vi "DeleteObstacle.vi"(6 "OldVal":bool, 7 "ID# To Delete (miss)":u16, 8 "error in (no error)":errorcluster, 10 "Obstacle Arrays Cluster IN":T1 {"Readable Obstacles"."Obstacle Array"."North" format="%#_10f"; "Readable Obstacles"."Obstacle Array"."East" format="%#_8f"}, 11 "NetworkStreamWriter in":refnum<class "NetworkStreamWriter.lvclass">) -> (0 "error out":errorcluster, 2 "Obstacle Arrays Cluster OUT":T1 {"Readable Obstacles"."Obstacle Array"."North" format="%#_10f"; "Readable Obstacles"."Obstacle Array"."East" format="%#_8f"}, 3 "NetworkStreamWriter out":refnum<class "NetworkStreamWriter.lvclass">)   [LabVIEW 2013]
doc: "This VI takes the \"ID to Delete\" value and\n1) Sends that ID down to the forebrain\n2) Deletes the objects with that ID from the OCU mission arrays\n\nEric Schneider, August 2014"
uses:
  RIO-OCU_Comm/NetworkStreams/Writer/NetworkStreamWriter.lvclass
  TypeDef/obstacle_arrays.ctl
  cRIO_Code/Logic/Classes/Obstacle/Obstacle.lvclass
  cRIO_Code/Data/TypeDefs/ObstacleDescription.ctl
  cRIO_Code/Data/TypeDefs/UTM Location.ctl
  CommandMessages.ctl
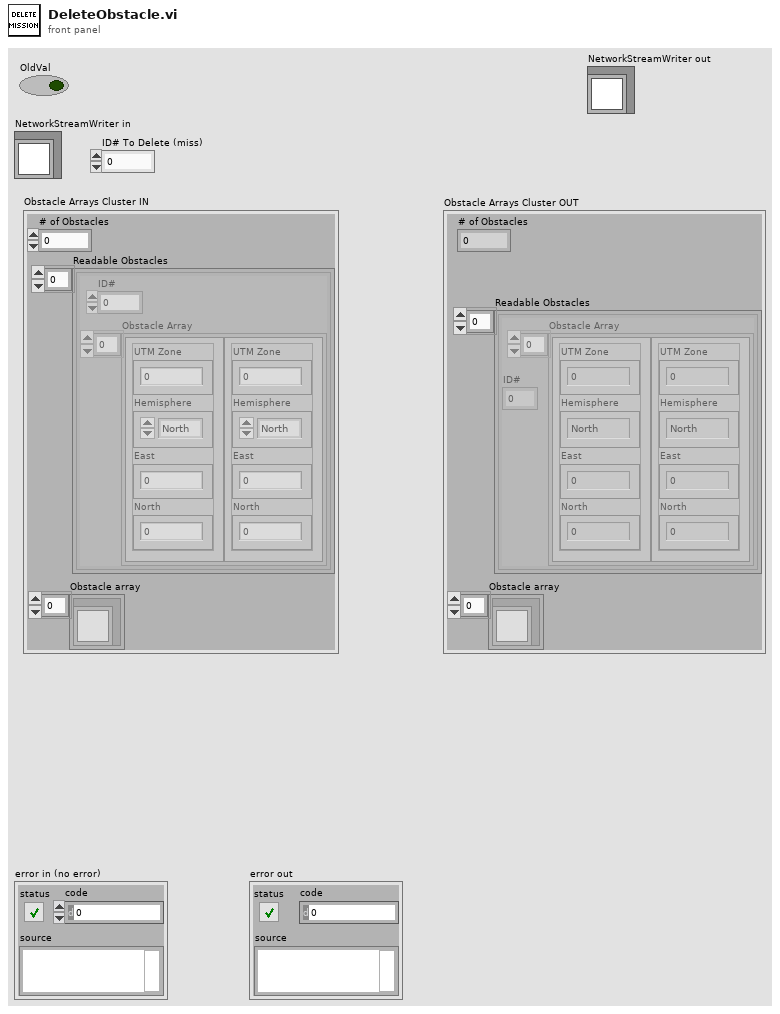
[diagram p1: front panel]
types:
  T1 = typedef "obstacle_arrays.ctl" = cluster{"# of Obstacles":i32, "Obstacle array":refnum<class "Obstacle.lvclass">[], "Readable Obstacles":T2[]}
  T2 = typedef "ObstacleDescription.ctl" = cluster{"ID#":i32, "Obstacle Array":T3[]}
  T3 = typedef "UTM Location.ctl" = cluster{"UTM Zone":dbl, "Hemisphere":enum16{"North", "South"}, "East":dbl, "North":dbl}
  T4 = typedef "CommandMessages.ctl" = enum16{"Pass", "OverrideMode", "Add mission", "Delete mission", "Add obstacle", "Delete obstacle", "Change constants"}
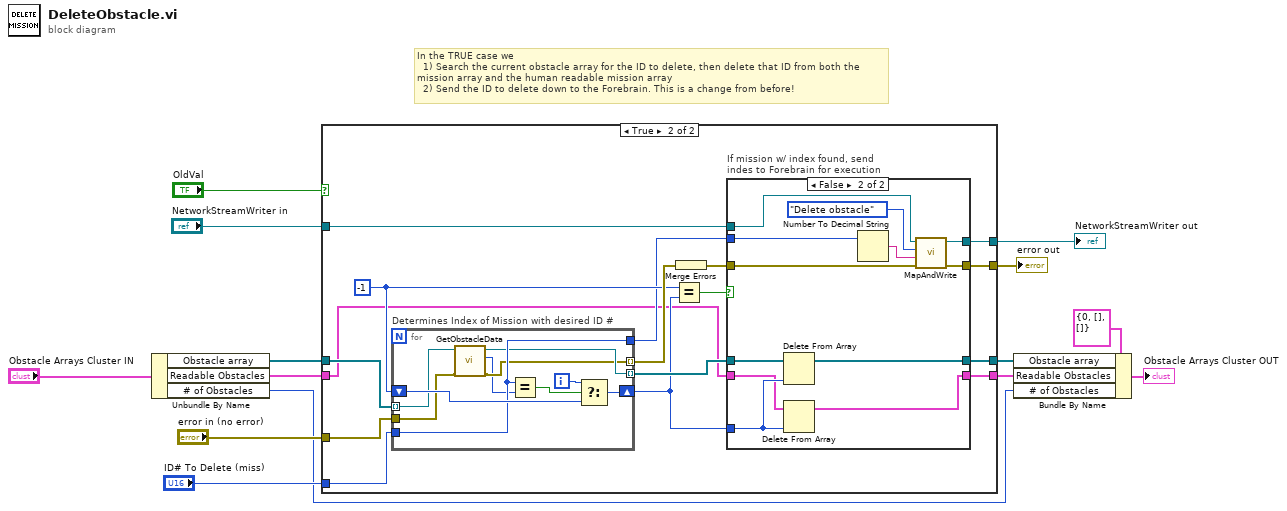
[diagram p0: block diagram]
diagram:
  # "In the TRUE case we\n  1) Search the current obstacle array for the ID to delete, then delete that ID from both the mission array and the human readable mission array\n  2) Send the ID to delete down to the Forebrain. This is a change from before!"
  n1 = Unbundle By Name("Obstacle Arrays Cluster IN") -> ("Obstacle array"=w10:refnum<class "Obstacle.lvclass">[], "Readable Obstacles"=w11:T2[], "# of Obstacles"=w1:i32)
  n2 = case shown="True" "OldVal" {
    tunnel: w10 -> [w15 w34]
    tunnel: [w15 w30] -> w12
    tunnel: [w16 w32] -> w13
    tunnel: [w17 w29] -> w6
    tunnel: "error in (no error)" -> [w17 w31]
    tunnel: "NetworkStreamWriter in" -> [w18 w24]
    tunnel: [w18 w28] -> w9
    tunnel: w11 -> [w16 w20]
    tunnel: "ID# To Delete (miss)" -> [_ w19]
    frame False {
    }
    frame True {
      w22 = -1
      n3 = for "Determines Index of Mission with desired ID #" {
        tunnel: w34 -> [w55] mode=indexing
        tunnel: [w54] -> w33 mode=indexing
        shift-right: [w58] -> w23
        shift-left: w22 -> [w57]
        tunnel: [w52] -> w26 mode=indexing
        tunnel: w31 -> [w53]
        tunnel: [w56] -> w21
        tunnel: w19 -> [w56]
        i -> [w59]
        n4 = call "GetObstacleData.vi"("error in (no error)"=w53, "Obstacle.lvclass"=w55) -> ("error out"=w52:errorcluster, "ID#"=w51:i32, "Obstacle"=w54:refnum<class "Obstacle.lvclass">)  [unwired: 6 in, 1 out]
        n5 = Equal?(x=w56, y=w51) -> (x = y?=w60:bool)
        n6 = Select(t=w59, s=w60, f=w57) -> (s? t:f=w58:i32)
      }
      n7 = Equal?(x=w22, y=w23) -> (x = y?=w27:bool)
      n8 = Merge Errors(w26) -> (w25:errorcluster)
      n9 = case "If mission w/ index found, send\nindes to Forebrain for execution" shown="False" w27 {
        tunnel: w33 -> [w36 w50]
        tunnel: [w35 w49] -> w32
        tunnel: w23 -> [_ w48]
        tunnel: w24 -> [w37 w47]
        tunnel: w25 -> [w38 w41]
        tunnel: [w36 w44] -> w30
        tunnel: [w38 w42] -> w29
        tunnel: [w37 w43] -> w28
        tunnel: w21 -> [_ w40]
        tunnel: w20 -> [w35 w39]
        frame True {
        }
        frame False {
          n10 = Delete From Array(array=w50, index=w48) -> (array with subset deleted=w44:refnum<class "Obstacle.lvclass">[])  [unwired: 1 in, 1 out]
          n11 = Delete From Array(array=w39, index=w48) -> (array with subset deleted=w49:T2[])  [unwired: 1 in, 1 out]
          n12 = Number To Decimal String(number=w40) -> (decimal integer string=w45:string)  [unwired: 1 in]
          n13 = call "MapAndWrite.vi"("error in (no error)"=w41, "String_Cast_of_Info"=w45, "Commands"=CommandMessages."Delete obstacle", "NetworkStreamWriter in"=w47) -> ("error out"=w42:errorcluster, "NetworkStreamWriter out"=w43:refnum<class "NetworkStreamWriter.lvclass">)  [unwired: 2 in]
        }
      }
    }
  }
  "NetworkStreamWriter out" <- w9
  "error out" <- w6
  n14 = Bundle By Name(cluster=T1 {"# of Obstacles"=0, "Obstacle array"=[], "Readable Obstacles"=[]} ("Obstacle Arrays Cluster IN"), "Obstacle array"=w12, "Readable Obstacles"=w13, "# of Obstacles"=w1) -> (→"Obstacle Arrays Cluster OUT":T1)
